vi "Add FPGA.vi"(6 "FPGA Target":T2, 8 "error in (no error)":errorcluster, 10 "Bitfile Path":path, 11 "Item Ref in":T1 format="%.0x") -> (0 "error out":errorcluster, 3 "Item Ref out":T1 format="%.0x")   [LabVIEW 2016, in "Scan Engine Custom Device.lvlib"]
uses:
  Scan Engine Custom Device.lvlib
  <vilib>/NI Veristand/Custom Device API/Custom Device Item Ref.ctl
  <vilib>/NI Veristand/Custom Device API/Custom Device API.lvlib
  Type Defs/FPGA Target.ctl
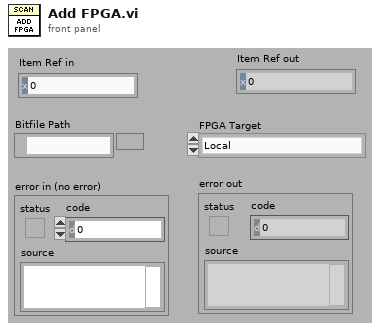
[diagram p1: front panel]
types:
  T1 = typedef "Custom Device API.lvlib/Custom Device Item Ref.ctl" = u64
  T2 = typedef "Scan Engine Custom Device.lvlib/FPGA Target.ctl" = enum16{"Local", "EtherCAT"}
  T3 = typedef "Scan Engine Custom Device.lvlib/Bitfile Signature.ctl" = cluster{"Signature (Hex) - Local FPGA":string, "Signature (SDO) - New ECAT API":u32, "Signature (XML) - Old ECAT API":u32}
  T4 = cluster{"name":string, "read":bool, "address":u32, "signed":bool, "size":u32, "datatype":string, "integersize":i32}[]
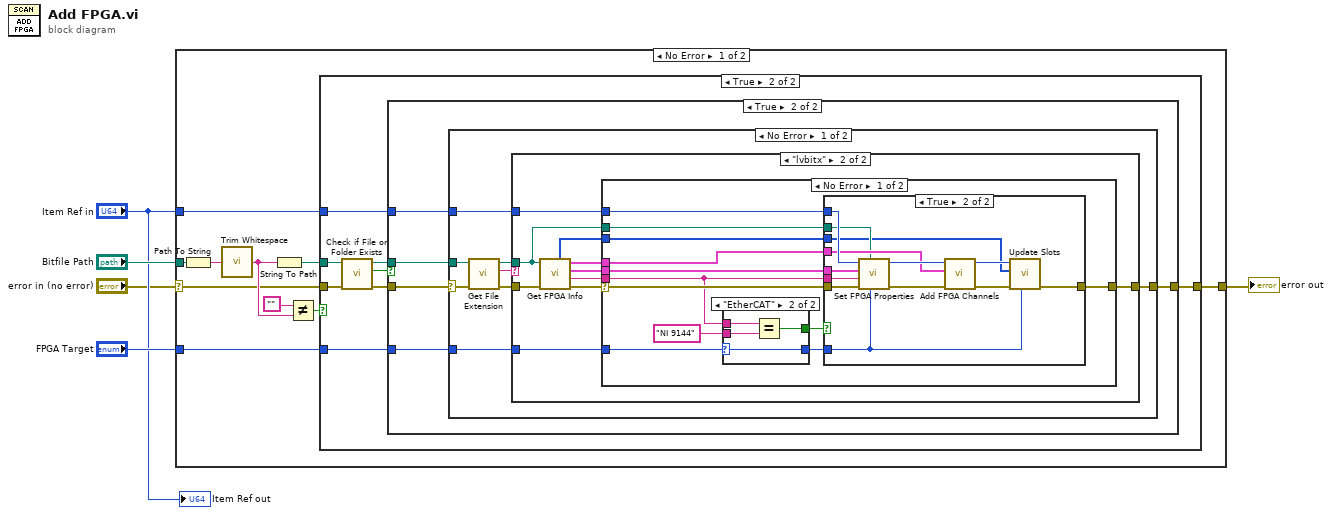
[diagram p0: block diagram]
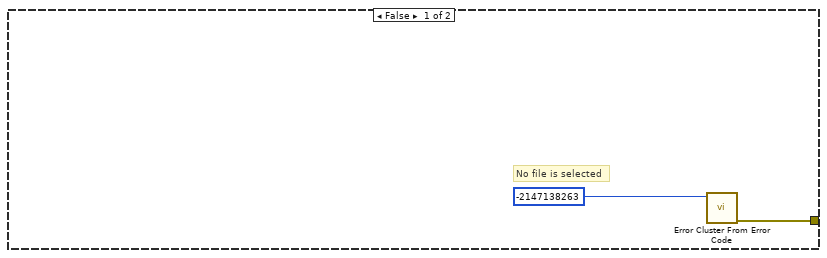
[diagram p2: hidden frame]
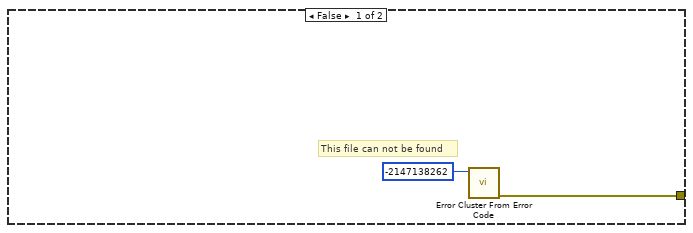
[diagram p3: hidden frame]
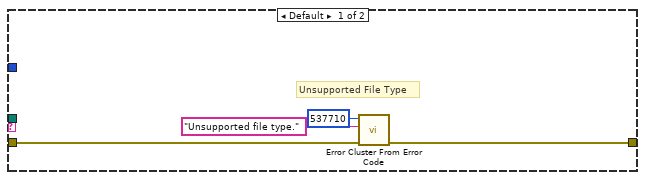
[diagram p4: hidden frame]
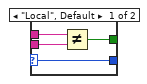
[diagram p5: hidden frame]
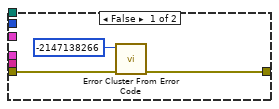
[diagram p6: hidden frame]
diagram:
  n1 = case shown="No Error" "error in (no error)" {
    selector: "error in (no error)" -> [w6 w93]
    tunnel: [w15 w93] -> w1
    tunnel: "Bitfile Path" -> [w14 _]
    tunnel: "FPGA Target" -> [w8 _]
    tunnel: "Item Ref in" -> [w7 _]
    frame No Error {
      n2 = Path To String(path=w14) -> (string=w11:string)
      n3 = call <vilib>:"Trim Whitespace.vi"("string"=w11) -> ("trimmed string"=w9:string)  [unwired: 1 in]
      n4 = String To Path(string=w9) -> (path=w13:path)
      n5 = Not Equal?(x="", y=w9) -> (x != y?=w12:bool)
      n6 = case shown="True" w12 {
        tunnel: w13 -> [_ w25]
        tunnel: [w16 w21] -> w15
        tunnel: w6 -> [_ w20]
        tunnel: w8 -> [_ w19]
        tunnel: w7 -> [_ w18]
        frame False {
          # "No file is selected"
          n7 = call <vilib>:"Error Cluster From Error Code.vi"("error code (0)"=-2147138263) -> ("error out"=w16:errorcluster)  [unwired: 8 in]
        }
        frame True {
          n8 = call <vilib>:"Check if File or Folder Exists.vi"("error in (no error)"=w20, "path"=w25) -> ("error out"=w23:errorcluster, "file or folder exists?"=w24:bool, "dup path"=w22:path)  [unwired: 7 out]
          n9 = case shown="True" w24 {
            tunnel: w23 -> [_ w31]
            tunnel: w22 -> [_ w32]
            tunnel: [w26 w30] -> w21
            tunnel: w19 -> [_ w29]
            tunnel: w18 -> [_ w28]
            frame False {
              # "This file can not be found"
              n10 = call <vilib>:"Error Cluster From Error Code.vi"("error code (0)"=-2147138262) -> ("error out"=w26:errorcluster)  [unwired: 8 in]
            }
            frame True {
              n11 = case shown="No Error" w31 {
                selector: w31 -> [w39 w92]
                tunnel: w32 -> [w40 _]
                tunnel: [w36 w92] -> w30
                tunnel: w29 -> [w34 _]
                tunnel: w28 -> [w33 _]
                frame No Error {
                  n12 = call <vilib>:"Get File Extension.vi"("error in (no error)"=w39, "file"=w40) -> ("error out"=w37:errorcluster, "lowercase file extension"=w38:string, "dup file"=w35:path)  [unwired: 7 out]
                  n13 = case shown="\"lvbitx\"" w38 {
                    tunnel: w37 -> [w44 w53]
                    tunnel: w35 -> [_ w47]
                    tunnel: [w43 w49] -> w36
                    tunnel: w34 -> [_ w48]
                    tunnel: w33 -> [_ w46]
                    frame Default {
                      # "Unsupported File Type"
                      n14 = call <vilib>:"Error Cluster From Error Code.vi"("error in (no error)"=w44, "error message (\"\")"="Unsupported file type." ("error message (\"\")"), "error code (0)"=537710) -> ("error out"=w43:errorcluster)  [unwired: 6 in]
                    }
                    frame "lvbitx" {
                      n15 = call "Get FPGA Info.vi"("error in"=w53, "Input bitfile path"=w47) -> ("error out"=w54:errorcluster, "TargetClass"=w52:string, "Signature"=w51:T3, "User defined IOVs"=w50:T4, "Scan Mode Slots"=w45:u32[])  [unwired: 5 in]
                      n16 = case shown="No Error" w54 {
                        selector: w54 -> [w64 w91]
                        tunnel: w52 -> [w60 _]
                        tunnel: w51 -> [w65 _]
                        tunnel: w50 -> [w66 _]
                        tunnel: [w63 w91] -> w49
                        tunnel: w48 -> [w59 _]
                        tunnel: w47 -> [w57 _]
                        tunnel: w46 -> [w56 _]
                        tunnel: w45 -> [w55 _]
                        frame No Error {
                          n17 = case shown="\"EtherCAT\"" w59 {
                            selector: w59 -> [w67 w71]
                            tunnel: [w70 w72] -> w62
                            tunnel: "NI 9144" ("y") -> [w69 w74]
                            tunnel: w60 -> [w68 w73]
                            tunnel: [w67 w71] -> w58
                            frame "Local", Default {
                              n18 = Not Equal?(x=w68, y=w69) -> (x != y?=w70:bool)
                            }
                            frame "EtherCAT" {
                              n19 = Equal?(x=w73, y=w74) -> (x = y?=w72:bool)
                            }
                          }
                          n20 = case shown="True" w62 {
                            tunnel: w66 -> [_ w84]
                            tunnel: w65 -> [_ w90]
                            tunnel: w64 -> [w76 w88]
                            tunnel: [w75 w81] -> w63
                            tunnel: w60 -> [_ w89]
                            tunnel: w58 -> [_ w78]
                            tunnel: w57 -> [_ w83]
                            tunnel: w56 -> [_ w87]
                            tunnel: w55 -> [_ w79]
                            frame False {
                              n21 = call <vilib>:"Error Cluster From Error Code.vi"("error in (no error)"=w76, "error code (0)"=-2147138266) -> ("error out"=w75:errorcluster)  [unwired: 7 in]
                            }
                            frame True {
                              n22 = call "Set FPGA Properties.vi"("FPGA Target"=w78, "Bitfile Path"=w83, "error in (no error)"=w88, "TargetClass"=w89, "Signature"=w90, "Item Ref in"=w87) -> ("error out"=w85:errorcluster, "Item Ref out"=w86:T1)  [unwired: 4 in]
                              n23 = call "Add FPGA Channels.vi"("error in (no error)"=w85, "User defined IOVs"=w84, "Item Ref in"=w86) -> ("error out"=w82:errorcluster, "Item Ref out"=w80:T1)  [unwired: 6 in]
                              n24 = call "Update Slots.vi"("FPGA Target"=w78, "error in (no error)"=w82, "Scan Mode Slots"=w79, "Item Ref in"=w80) -> ("error out"=w81:errorcluster)  [unwired: 6 in, 1 out]
                            }
                          }
                        }
                        frame Error {
                        }
                      }
                    }
                  }
                }
                frame Error {
                }
              }
            }
          }
        }
      }
    }
    frame Error {
    }
  }
  "error out" <- w1
  "Item Ref out" <- "Item Ref in"
